vi "Autonomous Independent.vi"   [LabVIEW 2016]
doc: "This VI is called when autonomous begins, and will automatically be terminated when autonomous ends. You can carry out timed or sensor driven robot movement independently without needing to return to the caller."
uses:
  <vilib>/Rock Robotics/WPI/Solenoid/WPI_SolenoidValue.ctl
  <vilib>/Rock Robotics/Network Tables/NT Read String.vi
  <vilib>/Rock Robotics/WPI/Utilities/WPI_GetSetVariantRefNum.vi
  <vilib>/Rock Robotics/WPI/Solenoid/WPI_SolenoidSetEnum.vi
  <vilib>/Rock Robotics/WPI/RobotDrive/WPI_RobotDriveArcadeDrive_Standard(NoSaturation).vi
panel:
  # "Be sure to right-click and choose Data Operations>>Make Current Value default if you want to save the array values with the VI"
types:
  T1 = typedef "WPI_SolenoidValue.ctl" = enum16{"Off", "On", "Forward", "Reverse"}
  T2 = typedef "WPI_SolenoidDevRef.ctl" = cluster{"DevStatus":errorcluster, "Pneumatics Control Module":u8, "Forward Solenoid Channel":T3, "Reverse Solenoid Channel":T3}
  T3 = typedef "WPI_SolenoidChannel.ctl" = enum8{"Solenoid 0", "Solenoid 1", "Solenoid 2", "Solenoid 3", "Solenoid 4", "Solenoid 5", "Solenoid 6", "Solenoid 7", "Invalid"}
  T4 = typedef "WPI_EncoderDevRef.ctl" = cluster{"DevStatus":errorcluster, "EncoderIndex":T5, "CounterIndex":T6, "DistancePerCount":dbl, "Decoding Type":T7}
  T5 = typedef "FPGA_EncoderIdx.ctl" = enum8{"Enc 0", "Enc 1", "Enc 2", "Enc 3", "Enc 4", "Enc 5", "Enc 6", "Enc 7", "Invalid"}
  T6 = typedef "FPGA_CounterCtrSystemIndex.ctl" = enum8{"Ctr 0", "Ctr 1", "Ctr 2", "Ctr 3", "Ctr 4", "Ctr 5", "Ctr 6", "Ctr 7", "Invalid"}
  T7 = typedef "WPI_EncoderType.ctl" = enum16{"1x", "2x", "4x"}
  T8 = typedef "WPI_MotorControlDeviceRef.ctl" = cluster{"DeviceStatus":errorcluster, "Type":T9, "PWM":cluster{"PWM Channel":T10, "DeadBand":T11}, "CAN":cluster{"Device Number":u8, "SetOutput VI Ref":variant, "GetOutput VI Ref":variant, "Enable VI Ref":variant, "Disable VI Ref":variant, "Data":variant}, "Invert":bool}
  T9 = typedef "WPI_MotorControlType.ctl" = enum16{"PWM", "CAN"}
  T10 = typedef "FPGA_DIOPWMChannel.ctl" = enum8{"PWM 0", "PWM 1", "PWM 2", "PWM 3", "PWM 4", "PWM 5", "PWM 6", "PWM 7", "PWM 8", "PWM 9", "PWM MXP 0", "PWM MXP 1", "PWM MXP 2", "PWM MXP 3", "PWM MXP 4", "PWM MXP 5", "PWM MXP 6", "PWM MXP 7", "PWM MXP 8", "PWM MXP 9", "Invalid"}
  T11 = typedef "WPI_PWMDeadband.ctl" = cluster{"Name":string, "maxPositivePwm":i32, "minPositivePwm":i32, "centerPwm":i32, "maxNegativePwm":i32, "minNegativePwm":i32, "angularRange":u16}
  T12 = typedef "WPI_RobotDriveDevRef.ctl" = cluster{"DevStatus":errorcluster, "Motors[]":T8[], "Square Inputs":bool, "Max Output":dbl}
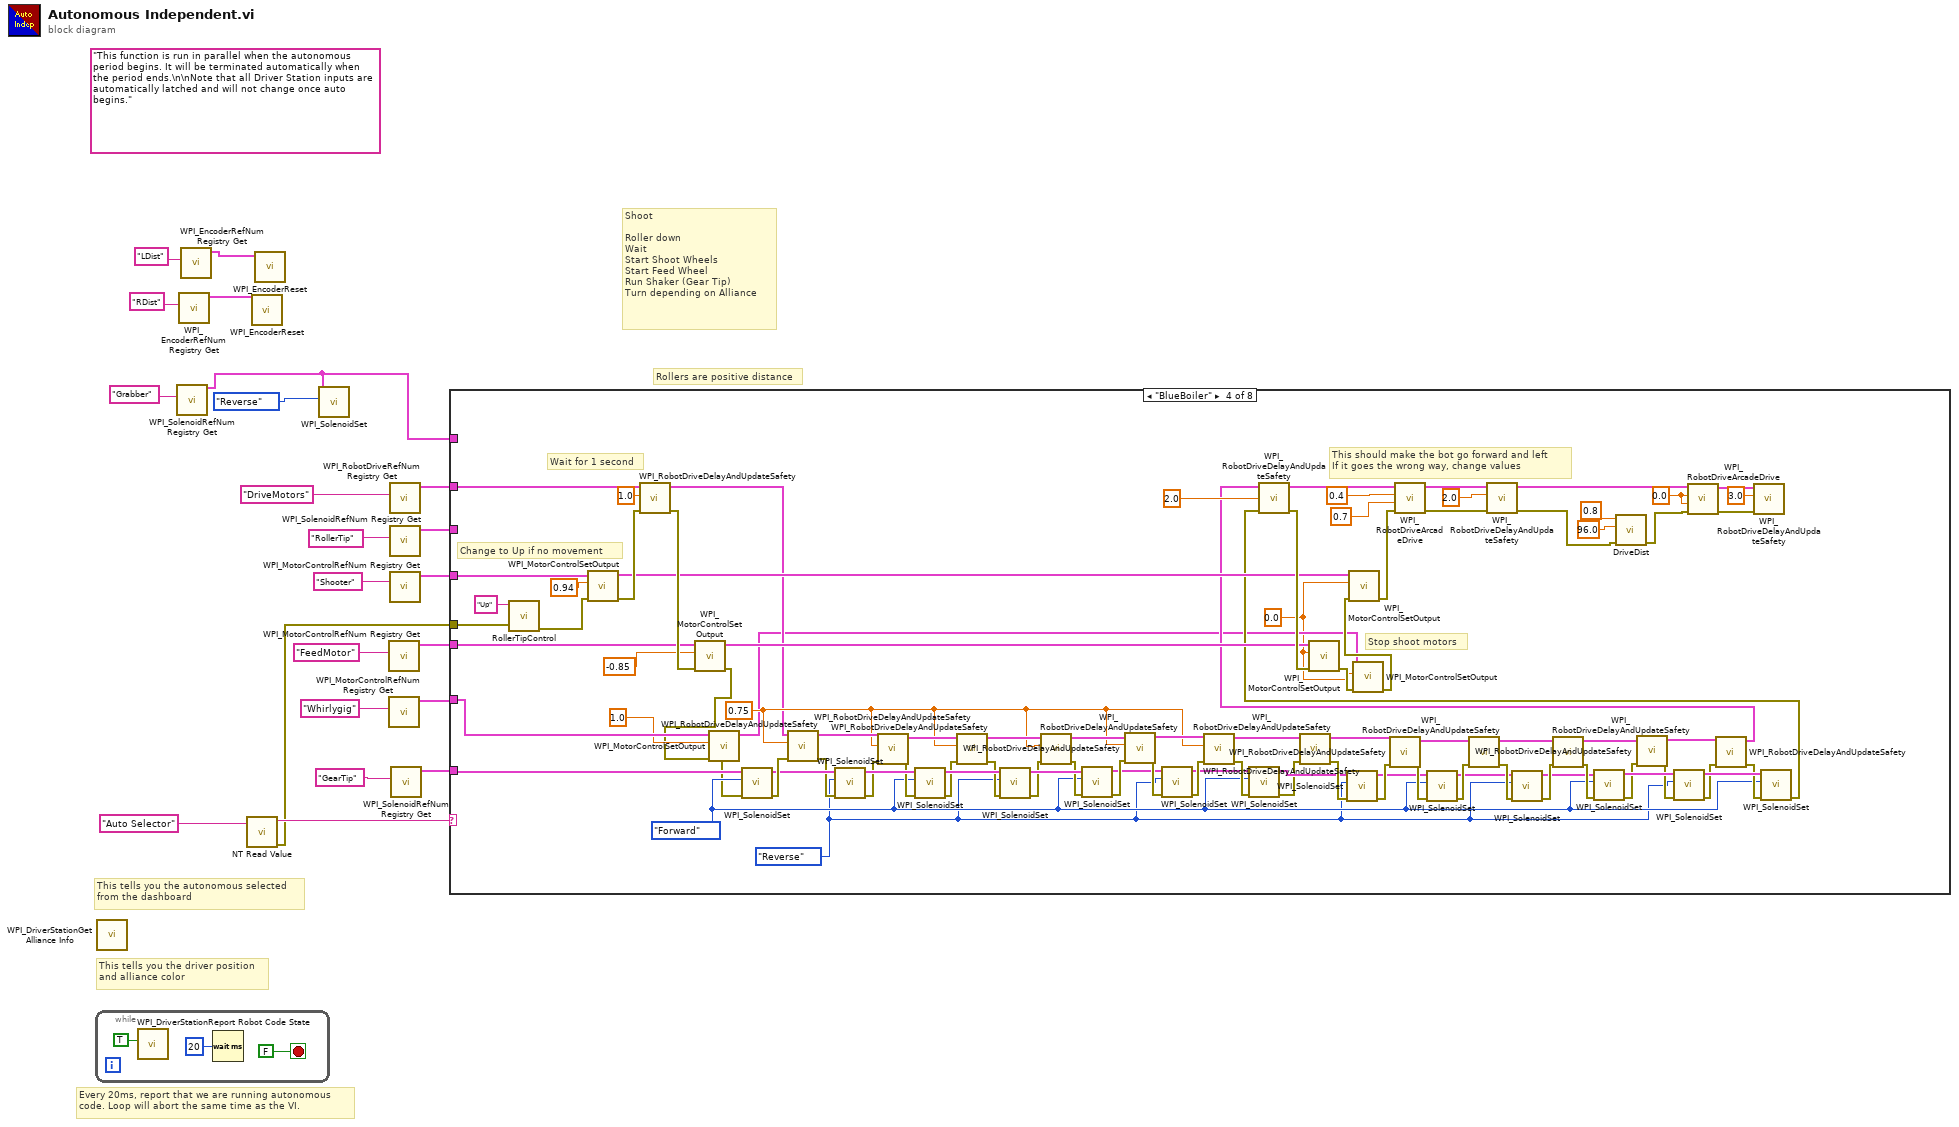
[diagram p0: block diagram]
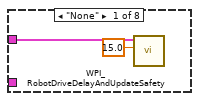
[diagram p2: hidden frame]
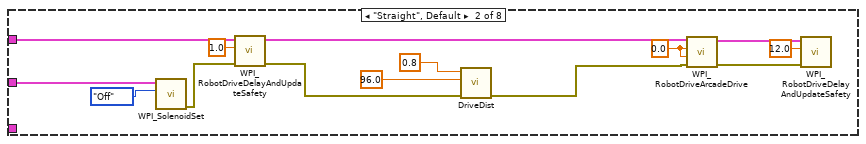
[diagram p3: hidden frame]
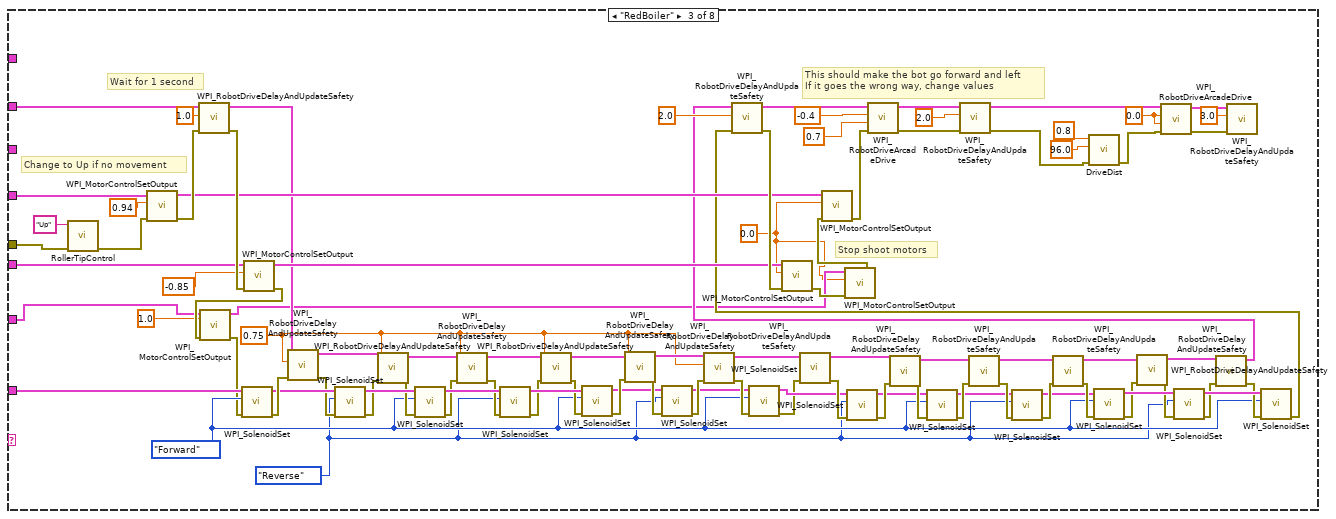
[diagram p4: hidden frame]
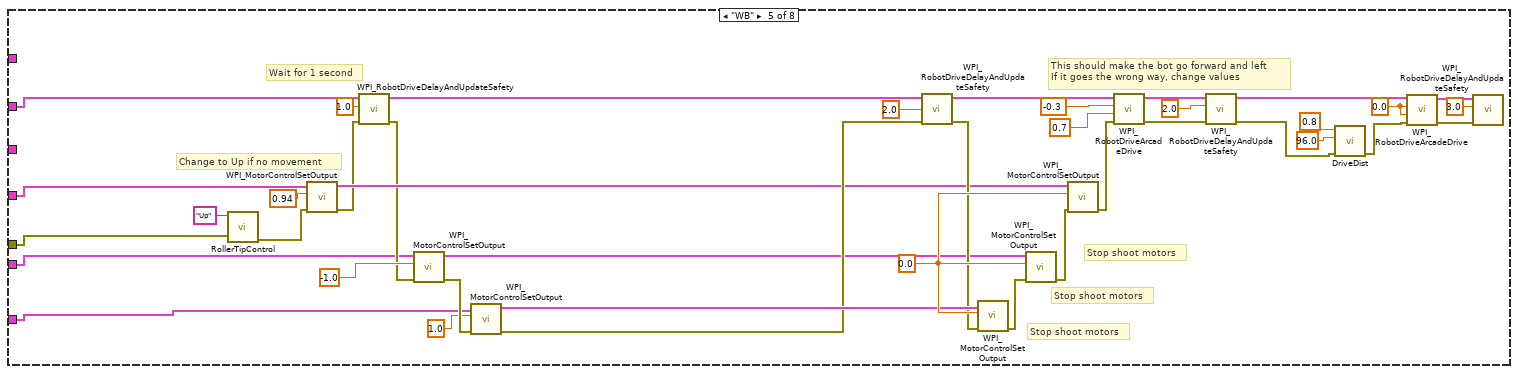
[diagram p5: hidden frame]
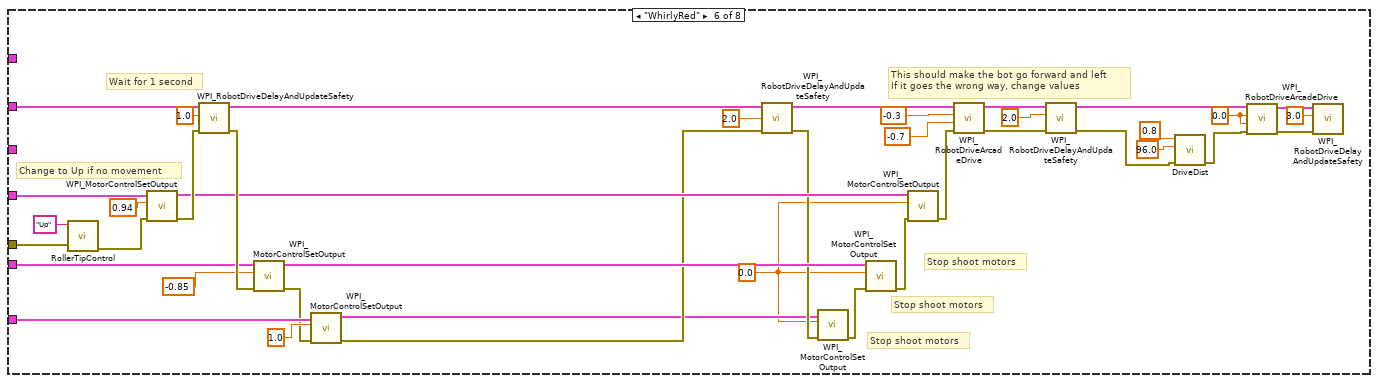
[diagram p6: hidden frame]
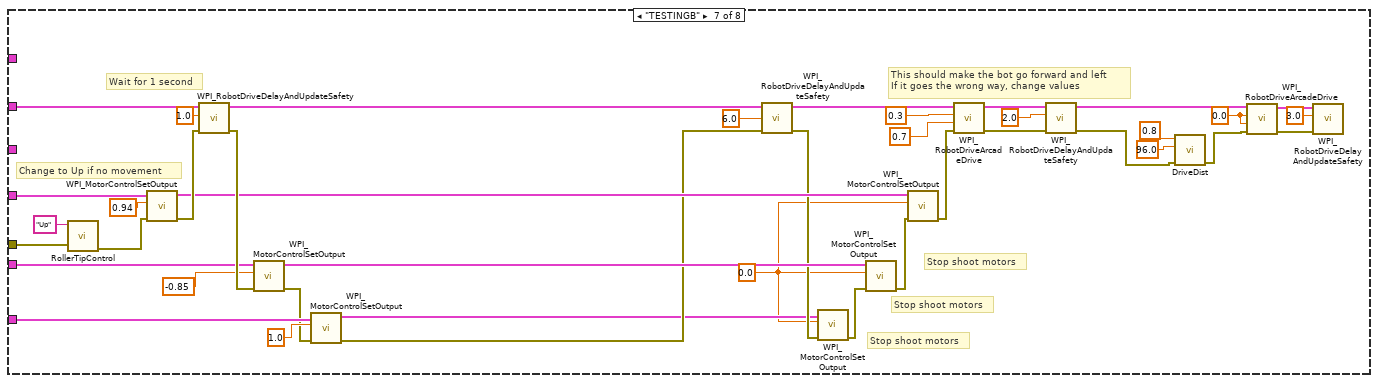
[diagram p7: hidden frame]
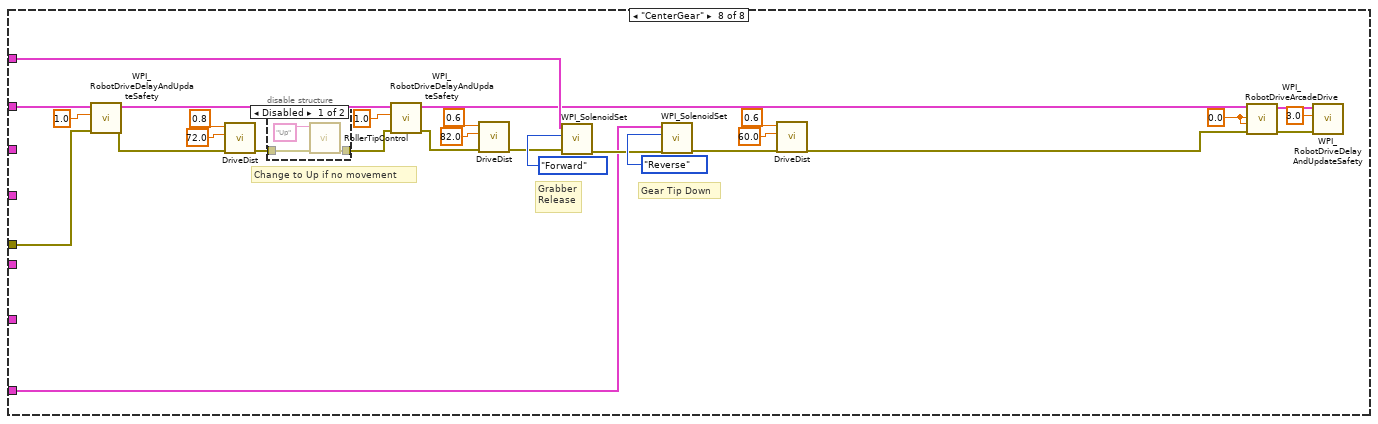
[diagram p8: hidden frame]
diagram:
  (unwired) "This function is run in parallel when the autonomous period begins. It will be terminated automatically when the period ends.\n\nNote that all Driver Station inputs are automatically latched and will not change once auto begins."
  # "Rollers are positive distance"
  # "Shoot\n\nRoller down \nWait\nStart Shoot Wheels      \nStart Feed Wheel\nRun Shaker (Gear Tip)\nTurn depending on Alliance"
  # "This tells you the autonomous selected\nfrom the dashboard"
  # "Every 20ms, report that we are running autonomous\ncode. Loop will abort the same time as the VI."
  # "This tells you the driver position\nand alliance color"
  n1 = while {
    stop <- FALSE stop-if-true
    n2 = call <vilib>:"WPI_DriverStationReport Robot Code State.vi"("Autonomous"=TRUE) -> ()  [unwired: 10 in, 1 out]
    n3 = Wait (ms)(milliseconds to wait=u32 20) -> ()  [unwired: 1 out]
  }
  n4 = call <vilib>:"WPI_DriverStationGet Alliance Info.vi"() -> ()  [unwired: 12 out]
  n5 = call <vilib>:"WPI_SolenoidRefNum Registry Get.vi"("refnum name"="Grabber") -> ("SolenoidDevRef"=w3:T2)  [unwired: 9 in, 1 out]
  n6 = call <vilib>:"WPI_EncoderRefNum Registry Get.vi"("refnum name"="RDist") -> ("EncoderDevRef"=w9:T4)  [unwired: 9 in, 1 out]
  n7 = call <vilib>:"WPI_EncoderRefNum Registry Get.vi"("refnum name"="LDist") -> ("EncoderDevRef"=w8:T4)  [unwired: 9 in, 1 out]
  n8 = call-poly <vilib>:"NT Read Value.vi"("Name"="Auto Selector") -> ("error out"=w12:errorcluster, "String"=w17:string)  [unwired: 9 in]
  n9 = call <vilib>:"WPI_EncoderReset.vi"("EncoderDevRef"=w9) -> ()  [unwired: 9 in, 2 out]
  n10 = call <vilib>:"WPI_EncoderReset.vi"("EncoderDevRef"=w8) -> ()  [unwired: 9 in, 2 out]
  n11 = call-poly <vilib>:"WPI_SolenoidSet.vi"("Value"=WPI_SolenoidValue."Reverse", "SolenoidDevRef"=w3) -> ()  [unwired: 8 in, 2 out]
  n12 = call <vilib>:"WPI_MotorControlRefNum Registry Get.vi"("refnum name"="FeedMotor") -> ("MotorControlDevRef"=w13:T8)  [unwired: 9 in, 1 out]
  n13 = call <vilib>:"WPI_MotorControlRefNum Registry Get.vi"("refnum name"="Whirlygig") -> ("MotorControlDevRef"=w1:T8)  [unwired: 9 in, 1 out]
  n14 = call <vilib>:"WPI_RobotDriveRefNum Registry Get.vi"("refnum name"="DriveMotors") -> ("RobotDriveDevRef"=w20:T12)  [unwired: 1 in, 9 out]
  n15 = call <vilib>:"WPI_SolenoidRefNum Registry Get.vi"("refnum name"="RollerTip") -> ("SolenoidDevRef"=w18:T2)  [unwired: 9 in, 1 out]
  n16 = call <vilib>:"WPI_MotorControlRefNum Registry Get.vi"("refnum name"="Shooter") -> ("MotorControlDevRef"=w14:T8)  [unwired: 9 in, 1 out]
  n17 = call <vilib>:"WPI_SolenoidRefNum Registry Get.vi"("refnum name"="GearTip") -> ("SolenoidDevRef"=w4:T2)  [unwired: 9 in, 1 out]
  n18 = case shown="\"BlueBoiler\"" w17 {
    tunnel: w20 -> [w27 w41 w134 w227 w228 w307 w347 w372]
    tunnel: w18 -> [_ w40 _ _ _ _ _ _]
    tunnel: w14 -> [_ _ w124 w217 w229 w297 w337 _]
    tunnel: w13 -> [_ _ w119 w212 w231 w292 w332 _]
    tunnel: w12 -> [_ _ w104 w143 w230 w278 w318 w368]
    tunnel: w4 -> [_ _ w103 w148 _ _ _ w354]
    tunnel: w1 -> [_ _ w46 w142 w232 w274 w314 _]
    tunnel: w3 -> [_ _ _ _ _ _ _ w357]
    frame "None" {
      n19 = call <vilib>:"WPI_RobotDriveDelayAndUpdateSafety.vi"("Delay (s)"=15.0, "RobotDriveDevRef"=w27) -> ()  [unwired: 8 in, 2 out]
    }
    frame "Straight", Default {
      w32 = 0.0 ("X axis value")
      n20 = call-poly <vilib>:"WPI_SolenoidSet.vi"("Value"=WPI_SolenoidValue."Off", "SolenoidDevRef"=w40) -> ("error out"=w37:errorcluster)  [unwired: 8 in, 1 out]
      n21 = call <vilib>:"WPI_RobotDriveDelayAndUpdateSafety.vi"("error in (no error)"=w37, "Delay (s)"=1.0, "RobotDriveDevRef"=w41) -> ("error out"=w36:errorcluster, "RobotDriveDevRef 2"=w33:T12)  [unwired: 7 in]
      n22 = call "DriveDist.vi"("error in (no error)"=w36, "DriveDist"=96.0, "saturation Dist"=0.8) -> ("error out"=w31:errorcluster)  [unwired: 8 in]
      n23 = call-poly <vilib>:"WPI_RobotDriveArcadeDrive.vi"("error in (no error)"=w31, "Y axis value"=w32, "X axis value"=w32, "RobotDriveDevRef"=w33) -> ("error out"=w30:errorcluster, "RobotDriveDevRef"=w29:T12)  [unwired: 5 in, 1 out]
      n24 = call <vilib>:"WPI_RobotDriveDelayAndUpdateSafety.vi"("error in (no error)"=w30, "Delay (s)"=12.0, "RobotDriveDevRef"=w29) -> ()  [unwired: 7 in, 2 out]
    }
    frame "RedBoiler" {
      w53 = WPI_SolenoidValue."Reverse" ("Value")
      w50 = 0.75 ("Delay (s)")
      w54 = WPI_SolenoidValue."Forward" ("Value")
      w42 = 0.0 ("Output")
      w130 = 0.0 ("X axis value")
      # "Change to Up if no movement"
      # "This should make the bot go forward and left\nIf it goes the wrong way, change values"
      # "Stop shoot motors"
      # "Wait for 1 second"
      n25 = call "RollerTipControl.vi"("error in (no error)"=w104, "Control"="Up") -> ("error out"=w122:errorcluster)  [unwired: 9 in]
      n26 = call <vilib>:"WPI_MotorControlSetOutput.vi"("error in (no error)"=w122, "Output"=0.94, "MotorControlDevRef"=w124) -> ("error out"=w121:errorcluster, "MotorControlDevRef"=w114:T8)  [unwired: 6 in, 1 out]
      n27 = call <vilib>:"WPI_RobotDriveDelayAndUpdateSafety.vi"("error in (no error)"=w121, "Delay (s)"=1.0, "RobotDriveDevRef"=w134) -> ("error out"=w120:errorcluster, "RobotDriveDevRef 2"=w102:T12)  [unwired: 7 in]
      n28 = call <vilib>:"WPI_MotorControlSetOutput.vi"("error in (no error)"=w120, "Output"=-0.85, "MotorControlDevRef"=w119) -> ("error out"=w49:errorcluster, "MotorControlDevRef"=w105:T8)  [unwired: 6 in, 1 out]
      n29 = call <vilib>:"WPI_MotorControlSetOutput.vi"("error in (no error)"=w49, "Output"=1.0, "MotorControlDevRef"=w46) -> ("error out"=w48:errorcluster, "MotorControlDevRef"=w43:T8)  [unwired: 6 in, 1 out]
      n30 = call-poly <vilib>:"WPI_SolenoidSet.vi"("error in (no error)"=w48, "Value"=w54, "SolenoidDevRef"=w103) -> ("error out"=w101:errorcluster, "SolenoidDevRef"=w100:T2)  [unwired: 7 in]
      n31 = call <vilib>:"WPI_RobotDriveDelayAndUpdateSafety.vi"("error in (no error)"=w101, "Delay (s)"=w50, "RobotDriveDevRef"=w102) -> ("error out"=w99:errorcluster, "RobotDriveDevRef 2"=w94:T12)  [unwired: 7 in]
      n32 = call-poly <vilib>:"WPI_SolenoidSet.vi"("error in (no error)"=w99, "Value"=w53, "SolenoidDevRef"=w100) -> ("error out"=w96:errorcluster, "SolenoidDevRef"=w98:T2)  [unwired: 7 in]
      n33 = call <vilib>:"WPI_RobotDriveDelayAndUpdateSafety.vi"("error in (no error)"=w96, "Delay (s)"=w50, "RobotDriveDevRef"=w94) -> ("error out"=w95:errorcluster, "RobotDriveDevRef 2"=w93:T12)  [unwired: 7 in]
      n34 = call-poly <vilib>:"WPI_SolenoidSet.vi"("error in (no error)"=w95, "Value"=w54, "SolenoidDevRef"=w98) -> ("error out"=w92:errorcluster, "SolenoidDevRef"=w97:T2)  [unwired: 7 in]
      n35 = call <vilib>:"WPI_RobotDriveDelayAndUpdateSafety.vi"("error in (no error)"=w92, "Delay (s)"=w50, "RobotDriveDevRef"=w93) -> ("error out"=w91:errorcluster, "RobotDriveDevRef 2"=w83:T12)  [unwired: 7 in]
      n36 = call-poly <vilib>:"WPI_SolenoidSet.vi"("error in (no error)"=w91, "Value"=w53, "SolenoidDevRef"=w97) -> ("error out"=w80:errorcluster, "SolenoidDevRef"=w81:T2)  [unwired: 7 in]
      n37 = call <vilib>:"WPI_RobotDriveDelayAndUpdateSafety.vi"("error in (no error)"=w80, "Delay (s)"=w50, "RobotDriveDevRef"=w83) -> ("error out"=w79:errorcluster, "RobotDriveDevRef 2"=w82:T12)  [unwired: 7 in]
      n38 = call-poly <vilib>:"WPI_SolenoidSet.vi"("error in (no error)"=w79, "Value"=w54, "SolenoidDevRef"=w81) -> ("error out"=w86:errorcluster, "SolenoidDevRef"=w84:T2)  [unwired: 7 in]
      n39 = call <vilib>:"WPI_RobotDriveDelayAndUpdateSafety.vi"("error in (no error)"=w86, "Delay (s)"=w50, "RobotDriveDevRef"=w82) -> ("error out"=w87:errorcluster, "RobotDriveDevRef 2"=w88:T12)  [unwired: 7 in]
      n40 = call-poly <vilib>:"WPI_SolenoidSet.vi"("error in (no error)"=w87, "Value"=w53, "SolenoidDevRef"=w84) -> ("error out"=w89:errorcluster, "SolenoidDevRef"=w85:T2)  [unwired: 7 in]
      n41 = call <vilib>:"WPI_RobotDriveDelayAndUpdateSafety.vi"("error in (no error)"=w89, "Delay (s)"=w50, "RobotDriveDevRef"=w88) -> ("error out"=w90:errorcluster, "RobotDriveDevRef 2"=w55:T12)  [unwired: 7 in]
      n42 = call-poly <vilib>:"WPI_SolenoidSet.vi"("error in (no error)"=w90, "Value"=w54, "SolenoidDevRef"=w85) -> ("error out"=w56:errorcluster, "SolenoidDevRef"=w57:T2)  [unwired: 7 in]
      n43 = call <vilib>:"WPI_RobotDriveDelayAndUpdateSafety.vi"("error in (no error)"=w56, "RobotDriveDevRef"=w55) -> ("error out"=w58:errorcluster, "RobotDriveDevRef 2"=w63:T12)  [unwired: 8 in]
      n44 = call-poly <vilib>:"WPI_SolenoidSet.vi"("error in (no error)"=w58, "Value"=w53, "SolenoidDevRef"=w57) -> ("error out"=w61:errorcluster, "SolenoidDevRef"=w59:T2)  [unwired: 7 in]
      n45 = call <vilib>:"WPI_RobotDriveDelayAndUpdateSafety.vi"("error in (no error)"=w61, "RobotDriveDevRef"=w63) -> ("error out"=w62:errorcluster, "RobotDriveDevRef 2"=w64:T12)  [unwired: 8 in]
      n46 = call-poly <vilib>:"WPI_SolenoidSet.vi"("error in (no error)"=w62, "Value"=w54, "SolenoidDevRef"=w59) -> ("error out"=w65:errorcluster, "SolenoidDevRef"=w60:T2)  [unwired: 7 in]
      n47 = call <vilib>:"WPI_RobotDriveDelayAndUpdateSafety.vi"("error in (no error)"=w65, "RobotDriveDevRef"=w64) -> ("error out"=w66:errorcluster, "RobotDriveDevRef 2"=w74:T12)  [unwired: 8 in]
      n48 = call-poly <vilib>:"WPI_SolenoidSet.vi"("error in (no error)"=w66, "Value"=w53, "SolenoidDevRef"=w60) -> ("error out"=w77:errorcluster, "SolenoidDevRef"=w76:T2)  [unwired: 7 in]
      n49 = call <vilib>:"WPI_RobotDriveDelayAndUpdateSafety.vi"("error in (no error)"=w77, "RobotDriveDevRef"=w74) -> ("error out"=w78:errorcluster, "RobotDriveDevRef 2"=w75:T12)  [unwired: 8 in]
      n50 = call-poly <vilib>:"WPI_SolenoidSet.vi"("error in (no error)"=w78, "Value"=w54, "SolenoidDevRef"=w76) -> ("error out"=w71:errorcluster, "SolenoidDevRef"=w73:T2)  [unwired: 7 in]
      n51 = call <vilib>:"WPI_RobotDriveDelayAndUpdateSafety.vi"("error in (no error)"=w71, "RobotDriveDevRef"=w75) -> ("error out"=w70:errorcluster, "RobotDriveDevRef 2"=w69:T12)  [unwired: 8 in]
      n52 = call-poly <vilib>:"WPI_SolenoidSet.vi"("error in (no error)"=w70, "Value"=w53, "SolenoidDevRef"=w73) -> ("error out"=w68:errorcluster, "SolenoidDevRef"=w72:T2)  [unwired: 7 in]
      n53 = call <vilib>:"WPI_RobotDriveDelayAndUpdateSafety.vi"("error in (no error)"=w68, "RobotDriveDevRef"=w69) -> ("error out"=w67:errorcluster, "RobotDriveDevRef 2"=w51:T12)  [unwired: 8 in]
      n54 = call-poly <vilib>:"WPI_SolenoidSet.vi"("error in (no error)"=w67, "Value"=w54, "SolenoidDevRef"=w72) -> ("error out"=w52:errorcluster)  [unwired: 7 in, 1 out]
      n55 = call <vilib>:"WPI_RobotDriveDelayAndUpdateSafety.vi"("error in (no error)"=w52, "Delay (s)"=2.0, "RobotDriveDevRef"=w51) -> ("error out"=w116:errorcluster, "RobotDriveDevRef 2"=w115:T12)  [unwired: 7 in]
      n56 = call <vilib>:"WPI_MotorControlSetOutput.vi"("error in (no error)"=w116, "Output"=w42, "MotorControlDevRef"=w105) -> ("error out"=w45:errorcluster)  [unwired: 6 in, 2 out]
      n57 = call <vilib>:"WPI_MotorControlSetOutput.vi"("error in (no error)"=w45, "Output"=w42, "MotorControlDevRef"=w43) -> ("error out"=w44:errorcluster)  [unwired: 6 in, 2 out]
      n58 = call <vilib>:"WPI_MotorControlSetOutput.vi"("error in (no error)"=w44, "Output"=w42, "MotorControlDevRef"=w114) -> ("error out"=w113:errorcluster)  [unwired: 6 in, 2 out]
      n59 = call-poly <vilib>:"WPI_RobotDriveArcadeDrive.vi"("error in (no error)"=w113, "Y axis value"=0.7, "X axis value"=-0.4, "RobotDriveDevRef"=w115) -> ("error out"=w107:errorcluster, "RobotDriveDevRef"=w109:T12)  [unwired: 5 in, 1 out]
      n60 = call <vilib>:"WPI_RobotDriveDelayAndUpdateSafety.vi"("error in (no error)"=w107, "Delay (s)"=2.0, "RobotDriveDevRef"=w109) -> ("error out"=w106:errorcluster, "RobotDriveDevRef 2"=w108:T12)  [unwired: 7 in]
      n61 = call "DriveDist.vi"("error in (no error)"=w106, "DriveDist"=96.0, "saturation Dist"=0.8) -> ("error out"=w129:errorcluster)  [unwired: 8 in]
      n62 = call-poly <vilib>:"WPI_RobotDriveArcadeDrive.vi"("error in (no error)"=w129, "Y axis value"=w130, "X axis value"=w130, "RobotDriveDevRef"=w108) -> ("error out"=w128:errorcluster, "RobotDriveDevRef"=w127:T12)  [unwired: 5 in, 1 out]
      n63 = call <vilib>:"WPI_RobotDriveDelayAndUpdateSafety.vi"("error in (no error)"=w128, "Delay (s)"=3.0, "RobotDriveDevRef"=w127) -> ()  [unwired: 7 in, 2 out]
    }
    frame "BlueBoiler" {
      w146 = 0.75 ("Delay (s)")
      w149 = WPI_SolenoidValue."Reverse" ("Value")
      w150 = WPI_SolenoidValue."Forward" ("Value")
      w135 = 0.0 ("Output")
      w223 = 0.0 ("X axis value")
      # "Change to Up if no movement"
      # "This should make the bot go forward and left\nIf it goes the wrong way, change values"
      # "Stop shoot motors"
      # "Wait for 1 second"
      n64 = call "RollerTipControl.vi"("error in (no error)"=w143, "Control"="Up") -> ("error out"=w215:errorcluster)  [unwired: 9 in]
      n65 = call <vilib>:"WPI_MotorControlSetOutput.vi"("error in (no error)"=w215, "Output"=0.94, "MotorControlDevRef"=w217) -> ("error out"=w214:errorcluster, "MotorControlDevRef"=w207:T8)  [unwired: 6 in, 1 out]
      n66 = call <vilib>:"WPI_RobotDriveDelayAndUpdateSafety.vi"("error in (no error)"=w214, "Delay (s)"=1.0, "RobotDriveDevRef"=w227) -> ("error out"=w213:errorcluster, "RobotDriveDevRef 2"=w145:T12)  [unwired: 7 in]
      n67 = call <vilib>:"WPI_MotorControlSetOutput.vi"("error in (no error)"=w213, "Output"=-0.85, "MotorControlDevRef"=w212) -> ("error out"=w140:errorcluster, "MotorControlDevRef"=w198:T8)  [unwired: 6 in, 1 out]
      n68 = call <vilib>:"WPI_MotorControlSetOutput.vi"("error in (no error)"=w140, "Output"=1.0, "MotorControlDevRef"=w142) -> ("error out"=w139:errorcluster, "MotorControlDevRef"=w136:T8)  [unwired: 6 in, 1 out]
      n69 = call-poly <vilib>:"WPI_SolenoidSet.vi"("error in (no error)"=w139, "Value"=w150, "SolenoidDevRef"=w148) -> ("error out"=w197:errorcluster, "SolenoidDevRef"=w196:T2)  [unwired: 7 in]
      n70 = call <vilib>:"WPI_RobotDriveDelayAndUpdateSafety.vi"("error in (no error)"=w197, "Delay (s)"=w146, "RobotDriveDevRef"=w145) -> ("error out"=w195:errorcluster, "RobotDriveDevRef 2"=w190:T12)  [unwired: 7 in]
      n71 = call-poly <vilib>:"WPI_SolenoidSet.vi"("error in (no error)"=w195, "Value"=w149, "SolenoidDevRef"=w196) -> ("error out"=w192:errorcluster, "SolenoidDevRef"=w194:T2)  [unwired: 7 in]
      n72 = call <vilib>:"WPI_RobotDriveDelayAndUpdateSafety.vi"("error in (no error)"=w192, "Delay (s)"=w146, "RobotDriveDevRef"=w190) -> ("error out"=w191:errorcluster, "RobotDriveDevRef 2"=w189:T12)  [unwired: 7 in]
      n73 = call-poly <vilib>:"WPI_SolenoidSet.vi"("error in (no error)"=w191, "Value"=w150, "SolenoidDevRef"=w194) -> ("error out"=w188:errorcluster, "SolenoidDevRef"=w193:T2)  [unwired: 7 in]
      n74 = call <vilib>:"WPI_RobotDriveDelayAndUpdateSafety.vi"("error in (no error)"=w188, "Delay (s)"=w146, "RobotDriveDevRef"=w189) -> ("error out"=w187:errorcluster, "RobotDriveDevRef 2"=w179:T12)  [unwired: 7 in]
      n75 = call-poly <vilib>:"WPI_SolenoidSet.vi"("error in (no error)"=w187, "Value"=w149, "SolenoidDevRef"=w193) -> ("error out"=w176:errorcluster, "SolenoidDevRef"=w177:T2)  [unwired: 7 in]
      n76 = call <vilib>:"WPI_RobotDriveDelayAndUpdateSafety.vi"("error in (no error)"=w176, "Delay (s)"=w146, "RobotDriveDevRef"=w179) -> ("error out"=w175:errorcluster, "RobotDriveDevRef 2"=w178:T12)  [unwired: 7 in]
      n77 = call-poly <vilib>:"WPI_SolenoidSet.vi"("error in (no error)"=w175, "Value"=w150, "SolenoidDevRef"=w177) -> ("error out"=w182:errorcluster, "SolenoidDevRef"=w180:T2)  [unwired: 7 in]
      n78 = call <vilib>:"WPI_RobotDriveDelayAndUpdateSafety.vi"("error in (no error)"=w182, "Delay (s)"=w146, "RobotDriveDevRef"=w178) -> ("error out"=w183:errorcluster, "RobotDriveDevRef 2"=w184:T12)  [unwired: 7 in]
      n79 = call-poly <vilib>:"WPI_SolenoidSet.vi"("error in (no error)"=w183, "Value"=w149, "SolenoidDevRef"=w180) -> ("error out"=w185:errorcluster, "SolenoidDevRef"=w181:T2)  [unwired: 7 in]
      n80 = call <vilib>:"WPI_RobotDriveDelayAndUpdateSafety.vi"("error in (no error)"=w185, "Delay (s)"=w146, "RobotDriveDevRef"=w184) -> ("error out"=w186:errorcluster, "RobotDriveDevRef 2"=w151:T12)  [unwired: 7 in]
      n81 = call-poly <vilib>:"WPI_SolenoidSet.vi"("error in (no error)"=w186, "Value"=w150, "SolenoidDevRef"=w181) -> ("error out"=w152:errorcluster, "SolenoidDevRef"=w153:T2)  [unwired: 7 in]
      n82 = call <vilib>:"WPI_RobotDriveDelayAndUpdateSafety.vi"("error in (no error)"=w152, "RobotDriveDevRef"=w151) -> ("error out"=w154:errorcluster, "RobotDriveDevRef 2"=w159:T12)  [unwired: 8 in]
      n83 = call-poly <vilib>:"WPI_SolenoidSet.vi"("error in (no error)"=w154, "Value"=w149, "SolenoidDevRef"=w153) -> ("error out"=w157:errorcluster, "SolenoidDevRef"=w155:T2)  [unwired: 7 in]
      n84 = call <vilib>:"WPI_RobotDriveDelayAndUpdateSafety.vi"("error in (no error)"=w157, "RobotDriveDevRef"=w159) -> ("error out"=w158:errorcluster, "RobotDriveDevRef 2"=w160:T12)  [unwired: 8 in]
      n85 = call-poly <vilib>:"WPI_SolenoidSet.vi"("error in (no error)"=w158, "Value"=w150, "SolenoidDevRef"=w155) -> ("error out"=w161:errorcluster, "SolenoidDevRef"=w156:T2)  [unwired: 7 in]
      n86 = call <vilib>:"WPI_RobotDriveDelayAndUpdateSafety.vi"("error in (no error)"=w161, "RobotDriveDevRef"=w160) -> ("error out"=w162:errorcluster, "RobotDriveDevRef 2"=w170:T12)  [unwired: 8 in]
      n87 = call-poly <vilib>:"WPI_SolenoidSet.vi"("error in (no error)"=w162, "Value"=w149, "SolenoidDevRef"=w156) -> ("error out"=w173:errorcluster, "SolenoidDevRef"=w172:T2)  [unwired: 7 in]
      n88 = call <vilib>:"WPI_RobotDriveDelayAndUpdateSafety.vi"("error in (no error)"=w173, "RobotDriveDevRef"=w170) -> ("error out"=w174:errorcluster, "RobotDriveDevRef 2"=w171:T12)  [unwired: 8 in]
      n89 = call-poly <vilib>:"WPI_SolenoidSet.vi"("error in (no error)"=w174, "Value"=w150, "SolenoidDevRef"=w172) -> ("error out"=w167:errorcluster, "SolenoidDevRef"=w169:T2)  [unwired: 7 in]
      n90 = call <vilib>:"WPI_RobotDriveDelayAndUpdateSafety.vi"("error in (no error)"=w167, "RobotDriveDevRef"=w171) -> ("error out"=w166:errorcluster, "RobotDriveDevRef 2"=w165:T12)  [unwired: 8 in]
      n91 = call-poly <vilib>:"WPI_SolenoidSet.vi"("error in (no error)"=w166, "Value"=w149, "SolenoidDevRef"=w169) -> ("error out"=w164:errorcluster, "SolenoidDevRef"=w168:T2)  [unwired: 7 in]
      n92 = call <vilib>:"WPI_RobotDriveDelayAndUpdateSafety.vi"("error in (no error)"=w164, "RobotDriveDevRef"=w165) -> ("error out"=w163:errorcluster, "RobotDriveDevRef 2"=w144:T12)  [unwired: 8 in]
      n93 = call-poly <vilib>:"WPI_SolenoidSet.vi"("error in (no error)"=w163, "Value"=w150, "SolenoidDevRef"=w168) -> ("error out"=w147:errorcluster)  [unwired: 7 in, 1 out]
      n94 = call <vilib>:"WPI_RobotDriveDelayAndUpdateSafety.vi"("error in (no error)"=w147, "Delay (s)"=2.0, "RobotDriveDevRef"=w144) -> ("error out"=w209:errorcluster, "RobotDriveDevRef 2"=w208:T12)  [unwired: 7 in]
      n95 = call <vilib>:"WPI_MotorControlSetOutput.vi"("error in (no error)"=w209, "Output"=w135, "MotorControlDevRef"=w198) -> ("error out"=w138:errorcluster)  [unwired: 6 in, 2 out]
      n96 = call <vilib>:"WPI_MotorControlSetOutput.vi"("error in (no error)"=w138, "Output"=w135, "MotorControlDevRef"=w136) -> ("error out"=w137:errorcluster)  [unwired: 6 in, 2 out]
      n97 = call <vilib>:"WPI_MotorControlSetOutput.vi"("error in (no error)"=w137, "Output"=w135, "MotorControlDevRef"=w207) -> ("error out"=w206:errorcluster)  [unwired: 6 in, 2 out]
      n98 = call-poly <vilib>:"WPI_RobotDriveArcadeDrive.vi"("error in (no error)"=w206, "Y axis value"=0.7, "X axis value"=0.4, "RobotDriveDevRef"=w208) -> ("error out"=w200:errorcluster, "RobotDriveDevRef"=w202:T12)  [unwired: 5 in, 1 out]
      n99 = call <vilib>:"WPI_RobotDriveDelayAndUpdateSafety.vi"("error in (no error)"=w200, "Delay (s)"=2.0, "RobotDriveDevRef"=w202) -> ("error out"=w199:errorcluster, "RobotDriveDevRef 2"=w201:T12)  [unwired: 7 in]
      n100 = call "DriveDist.vi"("error in (no error)"=w199, "DriveDist"=96.0, "saturation Dist"=0.8) -> ("error out"=w222:errorcluster)  [unwired: 8 in]
      n101 = call-poly <vilib>:"WPI_RobotDriveArcadeDrive.vi"("error in (no error)"=w222, "Y axis value"=w223, "X axis value"=w223, "RobotDriveDevRef"=w201) -> ("error out"=w221:errorcluster, "RobotDriveDevRef"=w220:T12)  [unwired: 5 in, 1 out]
      n102 = call <vilib>:"WPI_RobotDriveDelayAndUpdateSafety.vi"("error in (no error)"=w221, "Delay (s)"=3.0, "RobotDriveDevRef"=w220) -> ()  [unwired: 7 in, 2 out]
    }
    frame "WB" {
      w267 = 0.0 ("Output")
      w236 = 0.0 ("X axis value")
      # "Stop shoot motors"
      # "Stop shoot motors"
      # "Change to Up if no movement"
      # "This should make the bot go forward and left\nIf it goes the wrong way, change values"
      # "Stop shoot motors"
      # "Wait for 1 second"
      n103 = call "RollerTipControl.vi"("error in (no error)"=w230, "Control"="Up") -> ("error out"=w243:errorcluster)  [unwired: 9 in]
      n104 = call <vilib>:"WPI_MotorControlSetOutput.vi"("error in (no error)"=w243, "Output"=0.94, "MotorControlDevRef"=w229) -> ("error out"=w244:errorcluster, "MotorControlDevRef"=w249:T8)  [unwired: 6 in, 1 out]
      n105 = call <vilib>:"WPI_RobotDriveDelayAndUpdateSafety.vi"("error in (no error)"=w244, "Delay (s)"=1.0, "RobotDriveDevRef"=w228) -> ("error out"=w245:errorcluster, "RobotDriveDevRef 2"=w261:T12)  [unwired: 7 in]
      n106 = call <vilib>:"WPI_MotorControlSetOutput.vi"("error in (no error)"=w245, "Output"=-1.0, "MotorControlDevRef"=w231) -> ("error out"=w262:errorcluster, "MotorControlDevRef"=w258:T8)  [unwired: 6 in, 1 out]
      n107 = call <vilib>:"WPI_MotorControlSetOutput.vi"("error in (no error)"=w262, "Output"=1.0, "MotorControlDevRef"=w232) -> ("error out"=w263:errorcluster, "MotorControlDevRef"=w266:T8)  [unwired: 6 in, 1 out]
      n108 = call <vilib>:"WPI_RobotDriveDelayAndUpdateSafety.vi"("error in (no error)"=w263, "Delay (s)"=2.0, "RobotDriveDevRef"=w261) -> ("error out"=w264:errorcluster, "RobotDriveDevRef 2"=w248:T12)  [unwired: 7 in]
      n109 = call <vilib>:"WPI_MotorControlSetOutput.vi"("error in (no error)"=w264, "Output"=w267, "MotorControlDevRef"=w266) -> ("error out"=w265:errorcluster)  [unwired: 6 in, 2 out]
      n110 = call <vilib>:"WPI_MotorControlSetOutput.vi"("error in (no error)"=w265, "Output"=w267, "MotorControlDevRef"=w258) -> ("error out"=w247:errorcluster)  [unwired: 6 in, 2 out]
      n111 = call <vilib>:"WPI_MotorControlSetOutput.vi"("error in (no error)"=w247, "Output"=w267, "MotorControlDevRef"=w249) -> ("error out"=w250:errorcluster)  [unwired: 6 in, 2 out]
      n112 = call-poly <vilib>:"WPI_RobotDriveArcadeDrive.vi"("error in (no error)"=w250, "Y axis value"=0.7, "X axis value"=-0.3, "RobotDriveDevRef"=w248) -> ("error out"=w256:errorcluster, "RobotDriveDevRef"=w254:T12)  [unwired: 5 in, 1 out]
      n113 = call <vilib>:"WPI_RobotDriveDelayAndUpdateSafety.vi"("error in (no error)"=w256, "Delay (s)"=2.0, "RobotDriveDevRef"=w254) -> ("error out"=w257:errorcluster, "RobotDriveDevRef 2"=w255:T12)  [unwired: 7 in]
      n114 = call "DriveDist.vi"("error in (no error)"=w257, "DriveDist"=96.0, "saturation Dist"=0.8) -> ("error out"=w237:errorcluster)  [unwired: 8 in]
      n115 = call-poly <vilib>:"WPI_RobotDriveArcadeDrive.vi"("error in (no error)"=w237, "Y axis value"=w236, "X axis value"=w236, "RobotDriveDevRef"=w255) -> ("error out"=w238:errorcluster, "RobotDriveDevRef"=w239:T12)  [unwired: 5 in, 1 out]
      n116 = call <vilib>:"WPI_RobotDriveDelayAndUpdateSafety.vi"("error in (no error)"=w238, "Delay (s)"=3.0, "RobotDriveDevRef"=w239) -> ()  [unwired: 7 in, 2 out]
    }
    frame "WhirlyRed" {
      w268 = 0.0 ("Output")
      w303 = 0.0 ("X axis value")
      # "Stop shoot motors"
      # "Stop shoot motors"
      # "Change to Up if no movement"
      # "This should make the bot go forward and left\nIf it goes the wrong way, change values"
      # "Stop shoot motors"
      # "Wait for 1 second"
      n117 = call "RollerTipControl.vi"("error in (no error)"=w278, "Control"="Up") -> ("error out"=w295:errorcluster)  [unwired: 9 in]
      n118 = call <vilib>:"WPI_MotorControlSetOutput.vi"("error in (no error)"=w295, "Output"=0.94, "MotorControlDevRef"=w297) -> ("error out"=w294:errorcluster, "MotorControlDevRef"=w288:T8)  [unwired: 6 in, 1 out]
      n119 = call <vilib>:"WPI_RobotDriveDelayAndUpdateSafety.vi"("error in (no error)"=w294, "Delay (s)"=1.0, "RobotDriveDevRef"=w307) -> ("error out"=w293:errorcluster, "RobotDriveDevRef 2"=w275:T12)  [unwired: 7 in]
      n120 = call <vilib>:"WPI_MotorControlSetOutput.vi"("error in (no error)"=w293, "Output"=-0.85, "MotorControlDevRef"=w292) -> ("error out"=w273:errorcluster, "MotorControlDevRef"=w279:T8)  [unwired: 6 in, 1 out]
      n121 = call <vilib>:"WPI_MotorControlSetOutput.vi"("error in (no error)"=w273, "Output"=1.0, "MotorControlDevRef"=w274) -> ("error out"=w272:errorcluster, "MotorControlDevRef"=w269:T8)  [unwired: 6 in, 1 out]
      n122 = call <vilib>:"WPI_RobotDriveDelayAndUpdateSafety.vi"("error in (no error)"=w272, "Delay (s)"=2.0, "RobotDriveDevRef"=w275) -> ("error out"=w271:errorcluster, "RobotDriveDevRef 2"=w289:T12)  [unwired: 7 in]
      n123 = call <vilib>:"WPI_MotorControlSetOutput.vi"("error in (no error)"=w271, "Output"=w268, "MotorControlDevRef"=w269) -> ("error out"=w270:errorcluster)  [unwired: 6 in, 2 out]
      n124 = call <vilib>:"WPI_MotorControlSetOutput.vi"("error in (no error)"=w270, "Output"=w268, "MotorControlDevRef"=w279) -> ("error out"=w290:errorcluster)  [unwired: 6 in, 2 out]
      n125 = call <vilib>:"WPI_MotorControlSetOutput.vi"("error in (no error)"=w290, "Output"=w268, "MotorControlDevRef"=w288) -> ("error out"=w287:errorcluster)  [unwired: 6 in, 2 out]
      n126 = call-poly <vilib>:"WPI_RobotDriveArcadeDrive.vi"("error in (no error)"=w287, "Y axis value"=-0.7, "X axis value"=-0.3, "RobotDriveDevRef"=w289) -> ("error out"=w281:errorcluster, "RobotDriveDevRef"=w283:T12)  [unwired: 5 in, 1 out]
      n127 = call <vilib>:"WPI_RobotDriveDelayAndUpdateSafety.vi"("error in (no error)"=w281, "Delay (s)"=2.0, "RobotDriveDevRef"=w283) -> ("error out"=w280:errorcluster, "RobotDriveDevRef 2"=w282:T12)  [unwired: 7 in]
      n128 = call "DriveDist.vi"("error in (no error)"=w280, "DriveDist"=96.0, "saturation Dist"=0.8) -> ("error out"=w302:errorcluster)  [unwired: 8 in]
      n129 = call-poly <vilib>:"WPI_RobotDriveArcadeDrive.vi"("error in (no error)"=w302, "Y axis value"=w303, "X axis value"=w303, "RobotDriveDevRef"=w282) -> ("error out"=w301:errorcluster, "RobotDriveDevRef"=w300:T12)  [unwired: 5 in, 1 out]
      n130 = call <vilib>:"WPI_RobotDriveDelayAndUpdateSafety.vi"("error in (no error)"=w301, "Delay (s)"=3.0, "RobotDriveDevRef"=w300) -> ()  [unwired: 7 in, 2 out]
    }
    frame "TESTINGB" {
      w308 = 0.0 ("Output")
      w343 = 0.0 ("X axis value")
      # "Stop shoot motors"
      # "Stop shoot motors"
      # "Change to Up if no movement"
      # "This should make the bot go forward and left\nIf it goes the wrong way, change values"
      # "Stop shoot motors"
      # "Wait for 1 second"
      n131 = call "RollerTipControl.vi"("error in (no error)"=w318, "Control"="Up") -> ("error out"=w335:errorcluster)  [unwired: 9 in]
      n132 = call <vilib>:"WPI_MotorControlSetOutput.vi"("error in (no error)"=w335, "Output"=0.94, "MotorControlDevRef"=w337) -> ("error out"=w334:errorcluster, "MotorControlDevRef"=w328:T8)  [unwired: 6 in, 1 out]
      n133 = call <vilib>:"WPI_RobotDriveDelayAndUpdateSafety.vi"("error in (no error)"=w334, "Delay (s)"=1.0, "RobotDriveDevRef"=w347) -> ("error out"=w333:errorcluster, "RobotDriveDevRef 2"=w315:T12)  [unwired: 7 in]
      n134 = call <vilib>:"WPI_MotorControlSetOutput.vi"("error in (no error)"=w333, "Output"=-0.85, "MotorControlDevRef"=w332) -> ("error out"=w313:errorcluster, "MotorControlDevRef"=w319:T8)  [unwired: 6 in, 1 out]
      n135 = call <vilib>:"WPI_MotorControlSetOutput.vi"("error in (no error)"=w313, "Output"=1.0, "MotorControlDevRef"=w314) -> ("error out"=w312:errorcluster, "MotorControlDevRef"=w309:T8)  [unwired: 6 in, 1 out]
      n136 = call <vilib>:"WPI_RobotDriveDelayAndUpdateSafety.vi"("error in (no error)"=w312, "Delay (s)"=6.0, "RobotDriveDevRef"=w315) -> ("error out"=w311:errorcluster, "RobotDriveDevRef 2"=w329:T12)  [unwired: 7 in]
      n137 = call <vilib>:"WPI_MotorControlSetOutput.vi"("error in (no error)"=w311, "Output"=w308, "MotorControlDevRef"=w309) -> ("error out"=w310:errorcluster)  [unwired: 6 in, 2 out]
      n138 = call <vilib>:"WPI_MotorControlSetOutput.vi"("error in (no error)"=w310, "Output"=w308, "MotorControlDevRef"=w319) -> ("error out"=w330:errorcluster)  [unwired: 6 in, 2 out]
      n139 = call <vilib>:"WPI_MotorControlSetOutput.vi"("error in (no error)"=w330, "Output"=w308, "MotorControlDevRef"=w328) -> ("error out"=w327:errorcluster)  [unwired: 6 in, 2 out]
      n140 = call-poly <vilib>:"WPI_RobotDriveArcadeDrive.vi"("error in (no error)"=w327, "Y axis value"=0.7, "X axis value"=0.3, "RobotDriveDevRef"=w329) -> ("error out"=w321:errorcluster, "RobotDriveDevRef"=w323:T12)  [unwired: 5 in, 1 out]
      n141 = call <vilib>:"WPI_RobotDriveDelayAndUpdateSafety.vi"("error in (no error)"=w321, "Delay (s)"=2.0, "RobotDriveDevRef"=w323) -> ("error out"=w320:errorcluster, "RobotDriveDevRef 2"=w322:T12)  [unwired: 7 in]
      n142 = call "DriveDist.vi"("error in (no error)"=w320, "DriveDist"=96.0, "saturation Dist"=0.8) -> ("error out"=w342:errorcluster)  [unwired: 8 in]
      n143 = call-poly <vilib>:"WPI_RobotDriveArcadeDrive.vi"("error in (no error)"=w342, "Y axis value"=w343, "X axis value"=w343, "RobotDriveDevRef"=w322) -> ("error out"=w341:errorcluster, "RobotDriveDevRef"=w340:T12)  [unwired: 5 in, 1 out]
      n144 = call <vilib>:"WPI_RobotDriveDelayAndUpdateSafety.vi"("error in (no error)"=w341, "Delay (s)"=3.0, "RobotDriveDevRef"=w340) -> ()  [unwired: 7 in, 2 out]
    }
    frame "CenterGear" {
      w350 = 0.0
      # "Gear Tip Down"
      # "Grabber\nRelease"
      # "Change to Up if no movement"
      n145 = call <vilib>:"WPI_RobotDriveDelayAndUpdateSafety.vi"("error in (no error)"=w368, "Delay (s)"=1.0, "RobotDriveDevRef"=w372) -> ("error out"=w367:errorcluster, "RobotDriveDevRef 2"=w362:T12)  [unwired: 7 in]
      n146 = call "DriveDist.vi"("error in (no error)"=w367, "DriveDist"=72.0, "saturation Dist"=0.8) -> ("error out"=w366:errorcluster)  [unwired: 8 in]
      n147 = disable-structure shown="Disabled" {
        disable-tunnel: w366 -> [w377 _]
        disable-tunnel: [w376 _] -> w361
        frame Disabled {
          n148 = call "RollerTipControl.vi"("error in (no error)"=w377, "Control"="Up") -> ("error out"=w376:errorcluster)  [unwired: 9 in]
        }
        frame Enabled {
        }
      }
      n149 = call <vilib>:"WPI_RobotDriveDelayAndUpdateSafety.vi"("error in (no error)"=w361, "Delay (s)"=1.0, "RobotDriveDevRef"=w362) -> ("error out"=w360:errorcluster, "RobotDriveDevRef 2"=w349:T12)  [unwired: 7 in]
      n150 = call "DriveDist.vi"("error in (no error)"=w360, "DriveDist"=82.0, "saturation Dist"=0.6) -> ("error out"=w358:errorcluster)  [unwired: 8 in]
      n151 = call-poly <vilib>:"WPI_SolenoidSet.vi"("error in (no error)"=w358, "Value"=WPI_SolenoidValue."Forward", "SolenoidDevRef"=w357) -> ("error out"=w355:errorcluster)  [unwired: 7 in, 1 out]
      n152 = call-poly <vilib>:"WPI_SolenoidSet.vi"("error in (no error)"=w355, "Value"=WPI_SolenoidValue."Reverse", "SolenoidDevRef"=w354) -> ("error out"=w351:errorcluster)  [unwired: 7 in, 1 out]
      n153 = call "DriveDist.vi"("error in (no error)"=w351, "DriveDist"=60.0, "saturation Dist"=0.6) -> ("error out"=w348:errorcluster)  [unwired: 8 in]
      n154 = call-poly <vilib>:"WPI_RobotDriveArcadeDrive.vi"("error in (no error)"=w348, "Y axis value"=w350, "X axis value"=w350, "RobotDriveDevRef"=w349) -> ("error out"=w375:errorcluster, "RobotDriveDevRef"=w374:T12)  [unwired: 5 in, 1 out]
      n155 = call <vilib>:"WPI_RobotDriveDelayAndUpdateSafety.vi"("error in (no error)"=w375, "Delay (s)"=3.0, "RobotDriveDevRef"=w374) -> ()  [unwired: 7 in, 2 out]
    }
  }
